vi "FTW-Crypto-AES256.vi"(0 "Data":string="Data to encrypt!", 2 "Direction":enum16{"Encrypt", "Decrypt"}(ring), 5 "Key":string, 7 "Initialization Vector":string, 11 "error in":errorcluster) -> (4 "Data out":string, 6 "Key out":string, 8 "Initialization Vector out":string, 15 "error out":errorcluster)   [LabVIEW 2012]
uses:
  System.Core
panel:
  # "Inputs"
  # "Outputs"
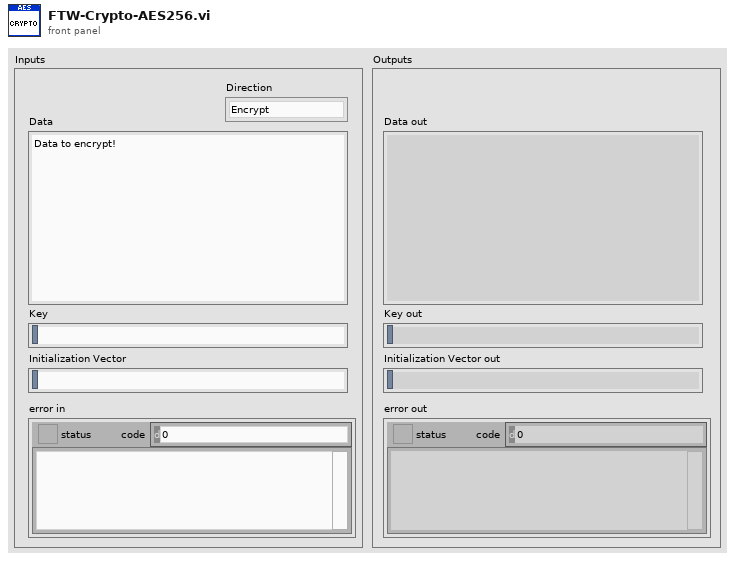
[diagram p1: front panel]
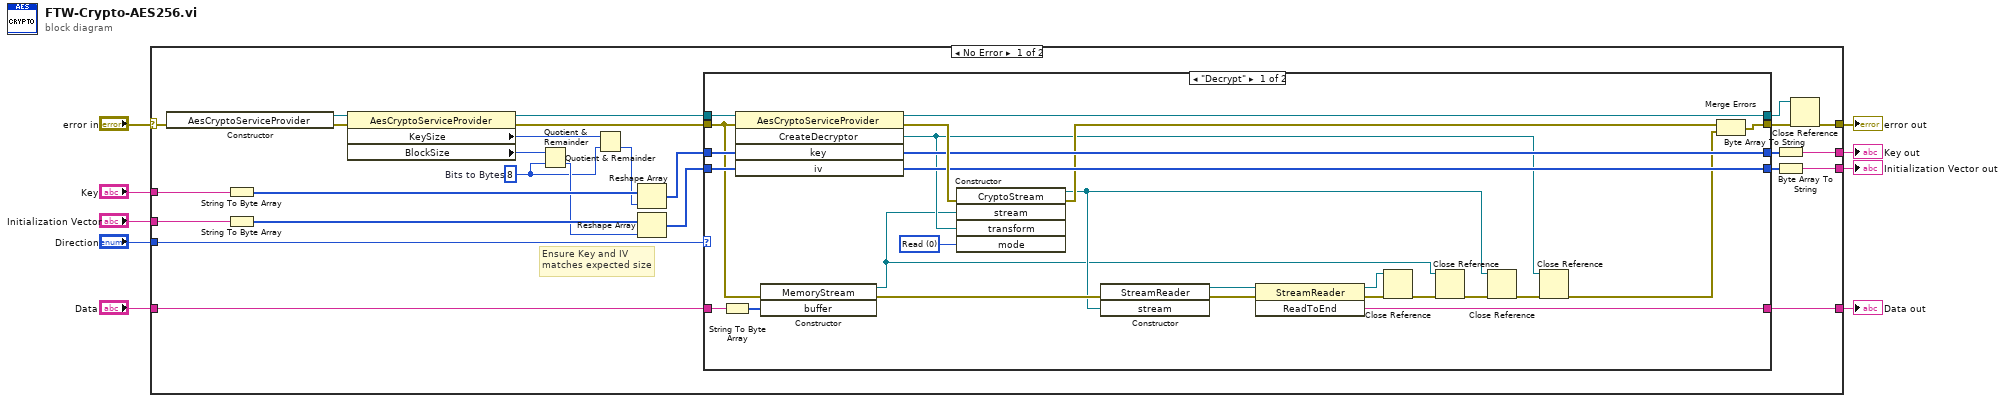
[diagram p0: block diagram]
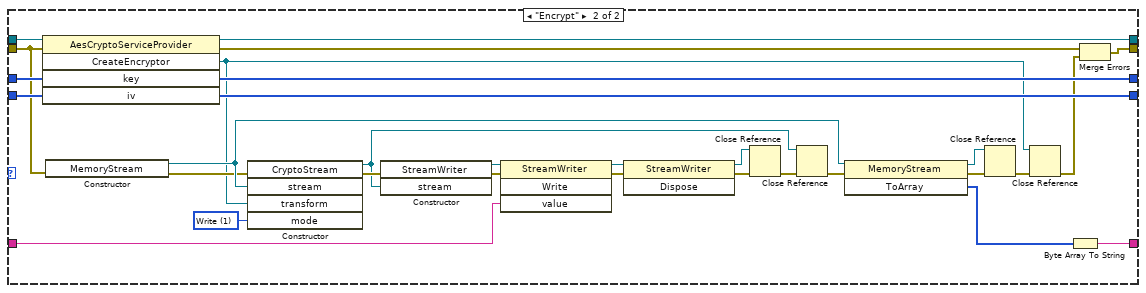
[diagram p2: hidden frame]
diagram:
  n1 = case shown="No Error" "error in" {
    selector: "error in" -> [w27 w95]
    tunnel: "Data" -> [w35 w94]
    tunnel: [w34 w92] -> w8
    tunnel: [w33 w93] -> w7
    tunnel: [w26 w94] -> w6
    tunnel: "Key" -> [w32 w93]
    tunnel: "Initialization Vector" -> [w31 w92]
    tunnel: "Direction" -> [w30 _]
    tunnel: [w23 w95] -> w1
    frame No Error {
      w10 = 8  # Bits to Bytes
      # "Ensure Key and IV\nmatches expected size"
      n2 = constructor class="AesCryptoServiceProvider"(error in=w27) -> (reference out=w22:refnum<k24>, error out=w21:errorcluster)  [unwired: 2 in, 1 out]
      n3 = String To Byte Array(string=w32) -> (unsigned byte array=w16:u8[])
      n4 = String To Byte Array(string=w31) -> (unsigned byte array=w18:u8[])
      n5 = property class="AesCryptoServiceProvider"(reference=w22, error in=w21) -> (reference out=w19:refnum<k24>, error out=w20:errorcluster, "KeySize"=w12:i32, "BlockSize"=w14:i32)
      n6 = Quotient & Remainder(x=w14, y=w10) -> (floor(x/y)=w13:i32)  [unwired: 1 out]
      n7 = Quotient & Remainder(x=w12, y=w10) -> (floor(x/y)=w11:i32)  [unwired: 1 out]
      n8 = Reshape Array(w16, w11) -> (w15:u8[])
      n9 = Reshape Array(w18, w13) -> (w17:u8[])
      n10 = case shown="\"Decrypt\"" w30 {
        tunnel: w35 -> [w56 w89]
        tunnel: w20 -> [w53 w74]
        tunnel: w19 -> [w54 w84]
        tunnel: w15 -> [w58 w80]
        tunnel: w17 -> [w57 w79]
        tunnel: [w50 w76] -> w29
        tunnel: [w49 w75] -> w28
        tunnel: [w51 w82] -> w26
        tunnel: [w45 w81] -> w25
        tunnel: [w48 w78] -> w24
        frame "Decrypt" {
          w61 = 0 items=["Read", "Write"] ("mode")
          n11 = String To Byte Array(string=w56) -> (unsigned byte array=w55:u8[])
          n12 = invoke class="AesCryptoServiceProvider" method="CreateDecryptor"(reference=w54, error in=w53, "key"=w58, "iv"=w57) -> (reference out=w48:refnum<k24>, error out=w52:errorcluster, "CreateDecryptor"=w41:refnum<k24>, "key"=w50:u8[], "iv"=w49:u8[])  [unwired: 1 in]
          n13 = constructor class="MemoryStream"(error in=w53, "buffer"=w55) -> (reference out=w36:refnum<k24>, error out=w47:errorcluster)  [unwired: 2 in, 2 out]
          n14 = constructor class="CryptoStream"(error in=w52, "stream"=w36, "transform"=w41, "mode"=w61) -> (reference out=w42:refnum<k24>, error out=w46:errorcluster)  [unwired: 2 in, 4 out]
          n15 = constructor class="StreamReader"(error in=w47, "stream"=w42) -> (reference out=w60:refnum<k24>, error out=w59:errorcluster)  [unwired: 2 in, 2 out]
          n16 = invoke class="StreamReader" method="ReadToEnd"(reference=w60, error in=w59) -> (reference out=w43:refnum<k24>, error out=w44:errorcluster, "ReadToEnd"=w51:string)  [unwired: 1 in]
          n17 = Close Reference(reference=w43, error in (no error)=w44) -> (error out=w38:errorcluster)
          n18 = Close Reference(reference=w36, error in (no error)=w38) -> (error out=w37:errorcluster)
          n19 = Close Reference(reference=w42, error in (no error)=w37) -> (error out=w40:errorcluster)
          n20 = Close Reference(reference=w41, error in (no error)=w40) -> (error out=w39:errorcluster)
          n21 = Merge Errors(w46, w39) -> (w45:errorcluster)
        }
        frame "Encrypt" {
          w91 = 1 items=["Read", "Write"] ("mode")
          n22 = invoke class="AesCryptoServiceProvider" method="CreateEncryptor"(reference=w84, error in=w74, "key"=w80, "iv"=w79) -> (reference out=w78:refnum<k24>, error out=w77:errorcluster, "CreateEncryptor"=w70:refnum<k24>, "key"=w76:u8[], "iv"=w75:u8[])  [unwired: 1 in]
          n23 = constructor class="MemoryStream"(error in=w74) -> (reference out=w88:refnum<k24>, error out=w87:errorcluster)  [unwired: 2 in, 1 out]
          n24 = constructor class="CryptoStream"(error in=w87, "stream"=w88, "transform"=w70, "mode"=w91) -> (reference out=w71:refnum<k24>, error out=w86:errorcluster)  [unwired: 2 in, 4 out]
          n25 = constructor class="StreamWriter"(error in=w86, "stream"=w71) -> (reference out=w90:refnum<k24>, error out=w85:errorcluster)  [unwired: 2 in, 2 out]
          n26 = invoke class="StreamWriter" method="Write"(reference=w90, error in=w85, "value"=w89) -> (reference out=w65:refnum<k24>, error out=w63:errorcluster)  [unwired: 1 in, 2 out]
          n27 = invoke class="StreamWriter" method="Dispose"(reference=w65, error in=w63) -> (reference out=w64:refnum<k24>, error out=w62:errorcluster)  [unwired: 1 in, 1 out]
          n28 = Close Reference(reference=w64, error in (no error)=w62) -> (error out=w69:errorcluster)
          n29 = Close Reference(reference=w71, error in (no error)=w69) -> (error out=w66:errorcluster)
          n30 = invoke class="MemoryStream" method="ToArray"(reference=w88, error in=w66) -> (reference out=w73:refnum<k24>, error out=w72:errorcluster, "ToArray"=w83:u8[])  [unwired: 1 in]
          n31 = Close Reference(reference=w73, error in (no error)=w72) -> (error out=w68:errorcluster)
          n32 = Close Reference(reference=w70, error in (no error)=w68) -> (error out=w67:errorcluster)
          n33 = Byte Array To String(unsigned byte array=w83) -> (string=w82:string)
          n34 = Merge Errors(w77, w67) -> (w81:errorcluster)
        }
      }
      n35 = Byte Array To String(unsigned byte array=w29) -> (string=w33:string)
      n36 = Byte Array To String(unsigned byte array=w28) -> (string=w34:string)
      n37 = Close Reference(reference=w24, error in (no error)=w25) -> (error out=w23:errorcluster)
    }
    frame Error {
    }
  }
  "Data out" <- w6
  "Initialization Vector out" <- w8
  "Key out" <- w7
  "error out" <- w1
